vi "Maquina_Contadora.vi"() -> ()   [LabVIEW 2016]
uses:
  Control3_Enum.ctl
panel:
  out "LED2":bool
  out "LED1":bool
  in  "Stop Button":bool
  in  "Boolean":bool
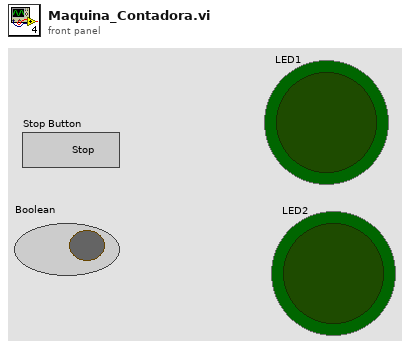
[diagram p1: front panel]
types:
  T1 = typedef "Control3_Enum.ctl" = enum16{"Caso 0", "Caso 1", "Caso 2", "Caso 3"}
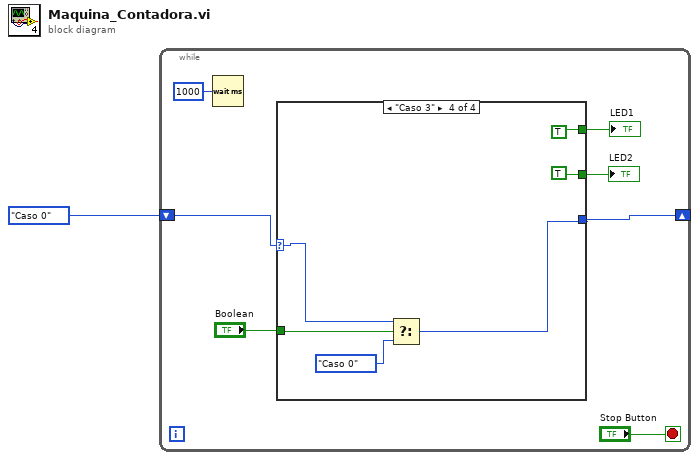
[diagram p0: block diagram]
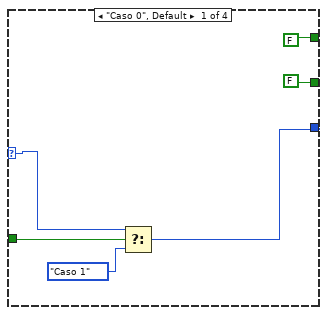
[diagram p2: hidden frame]
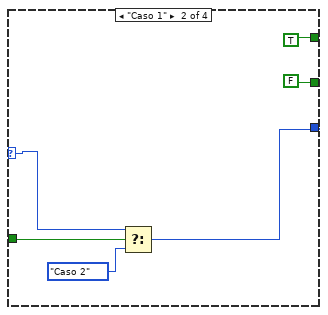
[diagram p3: hidden frame]
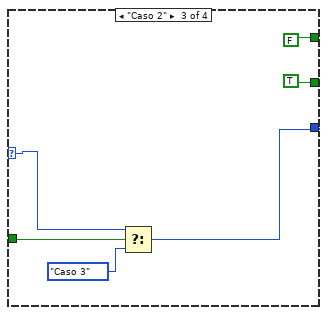
[diagram p4: hidden frame]
diagram:
  n1 = while {
    shift-right: [w6] -> _
    shift-left: Control3_Enum."Caso 0" -> [w8]
    stop <- "Stop Button" stop-if-true
    n2 = Wait (ms)(milliseconds to wait=u32 1000) -> ()  [unwired: 1 out]
    n3 = case shown="\"Caso 3\"" w8 {
      selector: w8 -> [w12 w18 w24 w30]
      tunnel: "Boolean" -> [w14 w20 w26 w32]
      tunnel: [w11 w17 w23 w29] -> w6
      tunnel: [FALSE FALSE TRUE TRUE] -> w4
      tunnel: [FALSE TRUE FALSE TRUE] -> w3
      frame "Caso 0", Default {
        n4 = Select(t=w12, s=w14, f=Control3_Enum."Caso 1") -> (s? t:f=w11:T1)
      }
      frame "Caso 1" {
        n5 = Select(t=w18, s=w20, f=Control3_Enum."Caso 2") -> (s? t:f=w17:T1)
      }
      frame "Caso 2" {
        n6 = Select(t=w24, s=w26, f=Control3_Enum."Caso 3") -> (s? t:f=w23:T1)
      }
      frame "Caso 3" {
        n7 = Select(t=w30, s=w32, f=Control3_Enum."Caso 0") -> (s? t:f=w29:T1)
      }
    }
    "LED1" <- w3
    "LED2" <- w4
  }
